vi "EventClient_RaiseEvent.vi"(6 "Top Priority":bool, 8 "error in (no error)":errorcluster, 10 "Data":variant, 11 "Event":string) -> (0 "error out":errorcluster)   [LabVIEW 2011]
uses:
  EventClient_ObjectReference.ctl
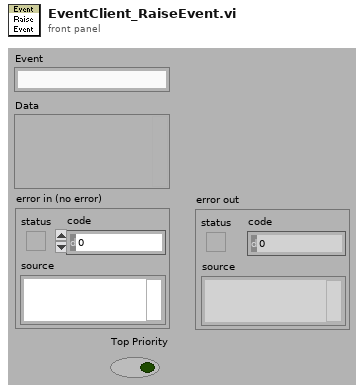
[diagram p1: front panel]
types:
  T1 = typedef "EventClient_ObjectReference.ctl" = refnum<k1>
  T2 = cluster{"Client":refnum<queue>, "Sub Events":string[], "PrvData":variant, "MyName":string}
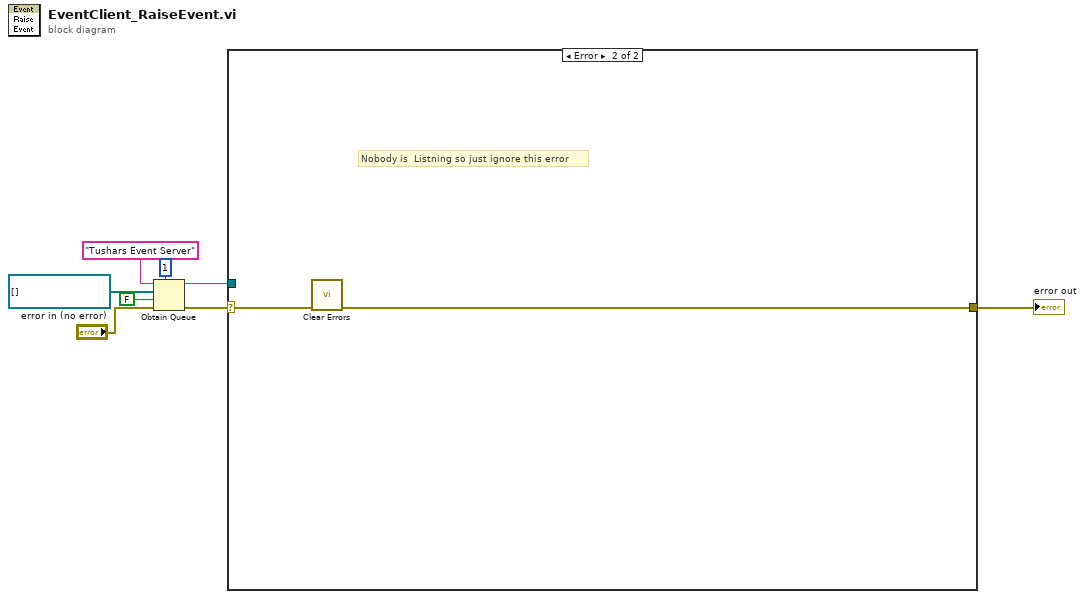
[diagram p0: block diagram]
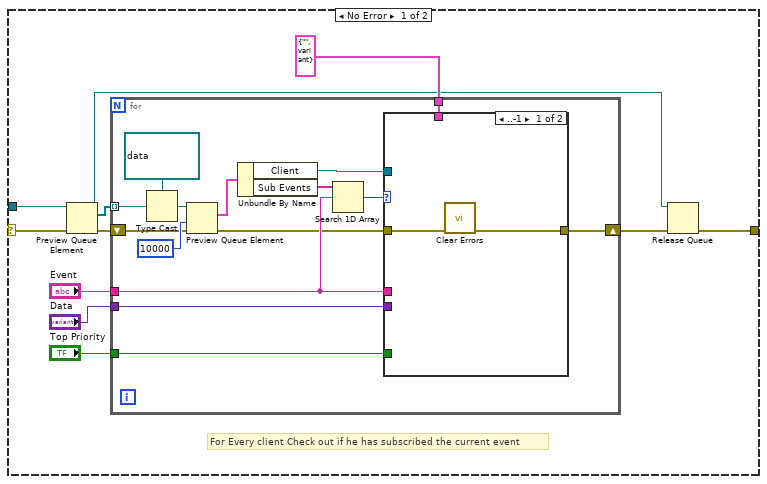
[diagram p2: hidden frame]
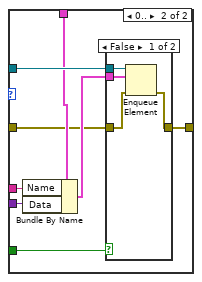
[diagram p3: hidden frame]
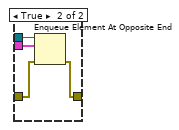
[diagram p4: hidden frame]
diagram:
  w5 = T1[] [] items=["EventClient"]
  n1 = Obtain Queue(max queue size (-1, unlimited)=1, name (unnamed)="Tushars Event Server", element data type=w5, create if not found? (T)=FALSE, error in (no error)="error in (no error)") -> (queue out=w7:refnum<queue>, error out=w1:errorcluster)  [unwired: 1 out]
  n2 = case shown="Error" w1 {
    selector: w1 -> [w9 w54]
    tunnel: w7 -> [w19 _]
    tunnel: [w11 w53] -> w2
    frame No Error {
      # "For Every client Check out if he has subscribed the current event"
      n3 = Preview Queue Element(queue=w19, error in (no error)=w9) -> (queue out=w10:refnum<queue>, element=w18:T1[], error out=w17:errorcluster)  [unwired: 2 out]
      n4 = for {
        tunnel: w18 -> [w34] mode=indexing
        shift-right: [w22] -> w12
        shift-left: w17 -> [w30]
        tunnel: "Event" -> [w24]
        tunnel: cluster{"Name":string, "Data":variant} {"Name"="", "Data"=variant} ("element") -> [w25]
        tunnel: "Data" -> [w23]
        tunnel: "Top Priority" -> [w20]
        n5 = Type Cast(type=refnum<queue> refnum ("queue out"), x=w34) -> (*(type *) &x=w33:refnum<queue>)
        n6 = Preview Queue Element(queue=w33, timeout in ms (-1)=10000, error in (no error)=w30) -> (element=w32:T2, error out=w21:errorcluster)  [unwired: 2 out]
        n7 = Unbundle By Name(w32) -> ("Client"=w26:refnum<queue>, "Sub Events"=w28:string[])
        n8 = Search 1D Array(1D array=w28, element=w24) -> (index of element=w27:i32)  [unwired: 1 out]
        n9 = case shown="..-1" w27 {
          tunnel: w26 -> [_ w44]
          tunnel: w25 -> [_ w43]
          tunnel: w24 -> [_ w42]
          tunnel: w23 -> [_ w41]
          tunnel: [w35 w38] -> w22
          tunnel: w21 -> [w36 w39]
          tunnel: w20 -> [_ w37]
          frame ..-1 {
            n10 = call <vilib>:"Clear Errors.vi"("error in (no error)"=w36) -> ("error out"=w35:errorcluster)  [unwired: 6 out]
          }
          frame 0.. {
            n11 = Bundle By Name(cluster=w43, "Name"=w42, "Data"=w41) -> (w40:cluster{"Name":string, "Data":variant})
            n12 = case shown="False" w37 {
              tunnel: w44 -> [w48 w52]
              tunnel: w40 -> [w47 w51]
              tunnel: w39 -> [w46 w50]
              tunnel: [w45 w49] -> w38
              frame False {
                n13 = Enqueue Element(queue=w48, element=w47, error in (no error)=w46) -> (error out=w45:errorcluster)  [unwired: 3 out]
              }
              frame True {
                n14 = Enqueue Element At Opposite End(queue=w52, element=w51, error in (no error)=w50) -> (error out=w49:errorcluster)  [unwired: 3 out]
              }
            }
          }
        }
      }
      n15 = Release Queue(queue=w10, error in (no error)=w12) -> (error out=w11:errorcluster)  [unwired: 3 out]
    }
    frame Error {
      # "Nobody is  Listning so just ignore this error"
      n16 = call <vilib>:"Clear Errors.vi"("error in (no error)"=w54) -> ("error out"=w53:errorcluster)  [unwired: 6 out]
    }
  }
  "error out" <- w2
